vi "flip2DVectorArray.vi"(10 "Y Vector Component Array":dbl[][](array[numeric]), 11 "X Vector Component Array":dbl[][](array[numeric])) -> (2 "Y Vector Component":dbl[][](array[numeric]), 3 "X Vector Component":dbl[][](array[numeric]))   [LabVIEW 2015]
uses:
  <userlib>/_OpenG.lib/array/array.llb/Reverse 2D Array (DBL)__ogtk.vi
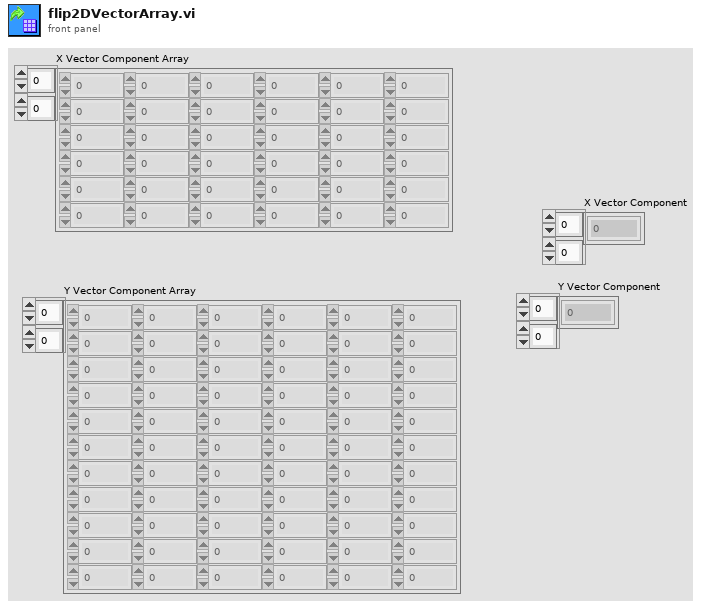
[diagram p1: front panel]
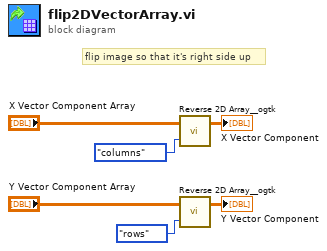
[diagram p0: block diagram]
diagram:
  # "flip image so that it's right side up"
  n1 = call-poly <userlib>:"Reverse 2D Array__ogtk.vi"("by rows or columns (rows)"=enum16{"rows", "columns"}."columns", "Array"="X Vector Component Array") -> ("Reversed Array"=→"X Vector Component":dbl[][])  [unwired: 1 in]
  n2 = call-poly <userlib>:"Reverse 2D Array__ogtk.vi"("by rows or columns (rows)"=enum16{"rows", "columns"}."rows", "Array"="Y Vector Component Array") -> ("Reversed Array"=→"Y Vector Component":dbl[][])  [unwired: 1 in]
